vi "Modbus Multi-Read U32.vi"(7 "Slave Address":u8, 8 "error in (no error)":errorcluster, 9 "Number of U32 to read":i32 format="%x", 10 "Register Start Address":u16 format="%x", 11 "VISA resource in":refnum<visa-resource-name>) -> (0 "error out":errorcluster, 1 "Output data [U32]":u32[](array[numeric]), 3 "VISA resource out":refnum<visa-resource-name>)   [LabVIEW 2024, in "Voegtlin_NI_SMART_Modbus_Drivers.lvlib"]
doc: "Lese die geforderte Anzahl U32-Werte ab der angegebenen Startadresse des selektierten Geraetes aus.\nDer COM-Port muss dazu initialisiert sein (benutze\" Modbus Init.vi\")."
uses:
  Voegtlin_NI_SMART_Modbus_Drivers.lvlib
  Enums/Modbus Comm.ctl
panel:
  out "Read register data\n U16 (array)":u16[](array[numeric])
  # "Input Data"
  # "Internal Data"
  # "Output Data"
  # "(Inputmaske in HEX)"
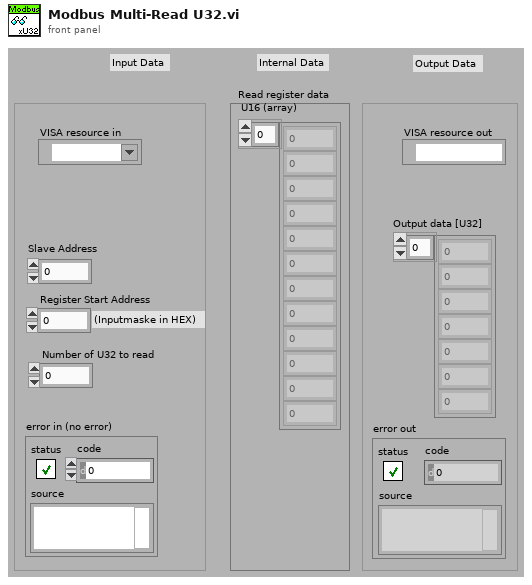
[diagram p1: front panel]
types:
  T1 = typedef "Voegtlin_NI_SMART_Modbus_Drivers.lvlib/Modbus Comm.ctl" = enum16{"Init", "Read", "Write", "Exit"}
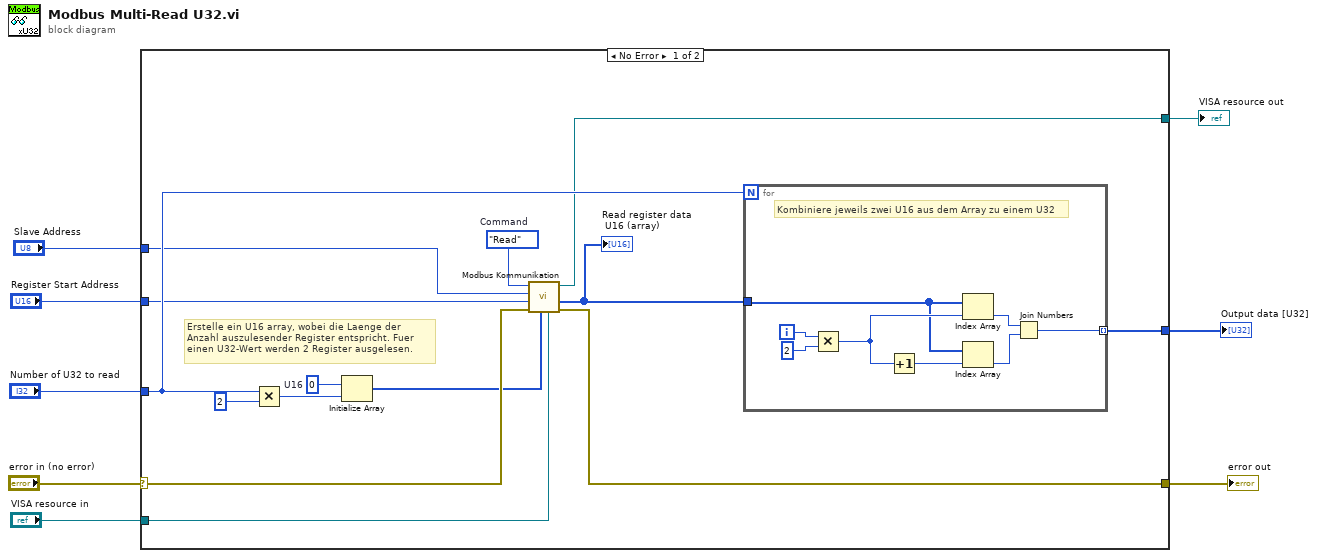
[diagram p0: block diagram]
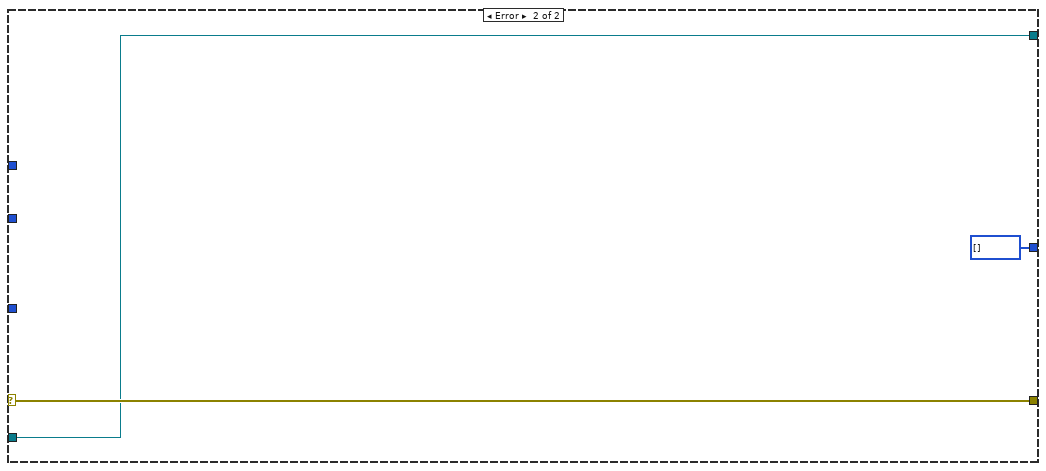
[diagram p2: hidden frame]
diagram:
  n1 = case shown="No Error" "error in (no error)" {
    selector: "error in (no error)" -> [w14 w33]
    tunnel: "Register Start Address" -> [w12 _]
    tunnel: [w22 w33] -> w7
    tunnel: "Number of U32 to read" -> [w17 _]
    tunnel: [w15 u32[] []] -> w5
    tunnel: "Slave Address" -> [w11 _]
    tunnel: "VISA resource in" -> [w10 w31]
    tunnel: [w9 w31] -> w1
    frame No Error {
      w20 = u16 0  # U16
      w21 = Modbus_Comm."Read"  # Command
      # "Erstelle ein U16 array, wobei die Laenge der Anzahl auszulesender Register entspricht. Fuer einen U32-Wert werden 2 Register ausgelesen."
      n2 = Multiply(x=w17, y=2) -> (x*y=w19:i32)
      n3 = Initialize Array(w20, w19) -> (w13:u16[])
      n4 = call "Modbus Kommunikation.vi"("VISA resource in"=w10, "Data In / #Reads [U16]"=w13, "error in (no error)"=w14, "Register Start Address"=w12, "Slave Address"=w11, "Command"=w21) -> ("error out"=w22:errorcluster, "Data Out [U16]"=w16:u16[], "VISA resource out"=w9:refnum<visa-resource-name>)  [unwired: 3 in]
      "Read register data\n U16 (array)" <- w16
      n5 = for {
        N: w17 -> [_]
        tunnel: w16 -> [w26]
        tunnel: [w23] -> w15 mode=indexing
        i -> [w29]
        # "Kombiniere jeweils zwei U16 aus dem Array zu einem U32"
        n6 = Multiply(x=w29, y=2 ("x")) -> (x*y=w28:i32)
        n7 = Increment(x=w28) -> (x+1=w27:i32)
        n8 = Index Array(array=w26, index=w28) -> (element=w25:u16)
        n9 = Index Array(array=w26, index=w27) -> (element=w24:u16)
        n10 = Join Numbers(hi=w25, lo=w24) -> ((hi.lo)=w23:u32)
      }
    }
    frame Error {
    }
  }
  "error out" <- w7
  "Output data [U32]" <- w5
  "VISA resource out" <- w1
